vi "Write Image.vi"(8 "error in (no error)":errorcluster, 10 "Matrix":T1[][](array[typedef]) items=["red"=0, "orange"=18, "yellow"=24, "green"=82, "cyan"=127, "blue"=170, "purple"=195, "pink"=220, "white"=254, "black"=255], 11 "I2C OLED in":refnum<class "RGB LED Matrix.lvclass">) -> (0 "error out":errorcluster, 3 "I2C OLED out":refnum<class "RGB LED Matrix.lvclass">)   [LabVIEW 2020, in "CTI-Peripheral.lvlib" / "RGB LED Matrix.lvclass"]
uses:
  RGB LED Matrix.lvclass
  Grove 2 RGB LED Matrix/Data Types/Colors.ctl
  Grove 2 RGB LED Matrix/Grove 2 RGB LED Matrix.lvclass
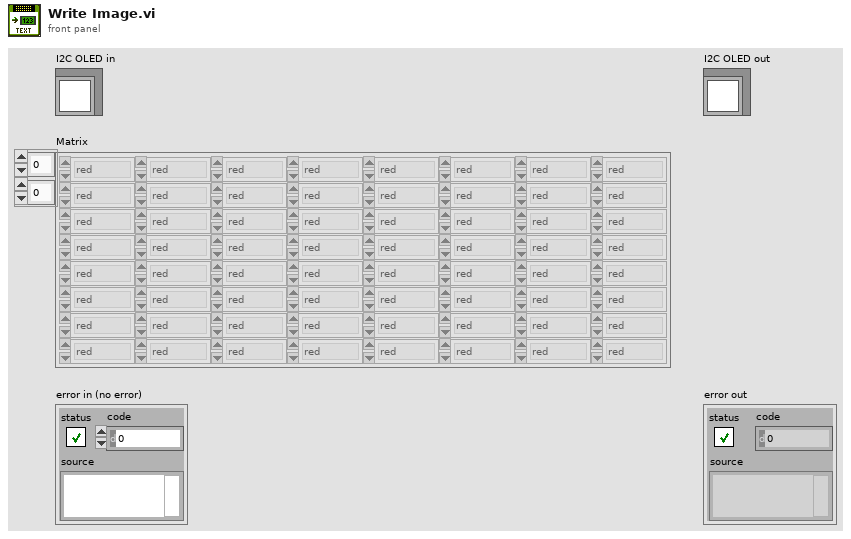
[diagram p1: front panel]
types:
  T1 = typedef "CTI-Peripheral.lvlib/Grove 2 RGB LED Matrix.lvclass/Colors.ctl" = u8
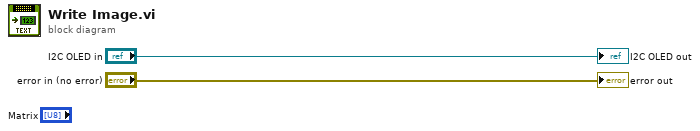
[diagram p0: block diagram]
diagram:
  "error out" <- "error in (no error)"
  "I2C OLED out" <- "I2C OLED in"
